vi "semLabV.vi"() -> ()   [LabVIEW 2021]
uses:
  <vilib>/userDefined/High Color/IMAQdx.ctl
  <vilib>/vision/driver/IMAQdx.llb/IMAQdx Camera Control Mode.ctl
  <vilib>/vision/driver/IMAQdx.llb/IMAQdx Acquisition Mode.ctl
  <vilib>/vision/driver/IMAQdx.llb/IMAQdx Buffer Number Mode.ctl
  <vilib>/myRIO/Instrument Drivers/Onboard IO/PWM/typedefs/PWM Reference.ctl
  <vilib>/myRIO/Common/Instrument Driver Framework/Utilities/typedefs/myRIO Generic Hardware Reference.ctl
  <vilib>/myRIO/Common/Instrument Driver Framework/Utilities/typedefs/Hardware Version Enum.ctl
  <vilib>/myRIO/Common/Instrument Driver Framework/Utilities/typedefs/myRIO v1.0 Reference.ctl
  <vilib>/myRIO/Common/Instrument Driver Framework/Utilities/typedefs/Generic FPGA Reference.ctl
  <vilib>/myRIO/Common/Instrument Driver Framework/myRIO v1.0/PWM/typedefs/PWM Channels Enum.ctl
  <vilib>/myRIO/Instrument Drivers/Onboard IO/PWM/typedefs/PWM Configuration.ctl
  <vilib>/userDefined/High Color/nirio_resource_hc.ctl
  <vilib>/myRIO/Common/Instrument Driver Framework/myRIO v1.0/PWM/vis/myRIO v1.1 Open PWM.vi
  <vilib>/myRIO/Common/Instrument Driver Framework/Utilities/vis/Validate Channels.vi
  <vilib>/myRIO/Common/Instrument Driver Framework/myRIO v1.0/PWM/vis/myRIO v1.0 Reserve PWM.vi
  <vilib>/myRIO/Instrument Drivers/Onboard IO/PWM/vis/Set Duty Cycle and Frequency.vi
  <vilib>/myRIO/Common/Instrument Driver Framework/myRIO v1.0/PWM/vis/myRIO v1.0 Close PWM.vi
  <vilib>/myRIO/Common/Instrument Driver Framework/myRIO v1.0/PWM/vis/myRIO v1.0 Build MUX Configuration PWM.vi
  <vilib>/myRIO/Common/Instrument Driver Framework/myRIO v1.0/Resource Manager/vis/myRIO v1.0 Reserve Channel List.vi
  <vilib>/myRIO/Common/Instrument Driver Framework/myRIO v1.0/PWM/vis/myRIO v1.0 Unreserve PWM.vi
  <vilib>/myRIO/Common/Instrument Driver Framework/myRIO v1.0/Resource Manager/vis/myRIO v1.0 Create Configuration List.vi
  <vilib>/myRIO/Common/Instrument Driver Framework/myRIO v1.0/Resource Manager/vis/myRIO v1.0 Reserve Channel.vi
  <vilib>/myRIO/Common/Instrument Driver Framework/myRIO v1.0/Resource Manager/vis/myRIO v1.0 Unreserve Channel.vi
  <vilib>/myRIO/Common/Instrument Driver Framework/myRIO v1.0/Resource Manager/vis/myRIO v1.0 Unreserve Channel List.vi
  <vilib>/myRIO/Common/Instrument Driver Framework/myRIO v1.0/Resource Manager/vis/myRIO v1.0 Build Mutex Name.vi
  <vilib>/Utility/VariantDataType/GetNumericInfo.vi
  <vilib>/Utility/error.llb/Error Cluster From Error Code.vi
  <vilib>/myRIO/Common/Instrument Driver Framework/myRIO v1.0/myRIO v1.1 Open.vi
  <vilib>/myRIO/Common/Instrument Driver Framework/Utilities/vis/IO Manager.vi
  <vilib>/myRIO/Common/Instrument Driver Framework/Utilities/vis/Configuration Manager.vi
  <vilib>/myRIO/Common/Instrument Driver Framework/myRIO v1.0/Resource Manager/vis/myRIO v1.0 Configure IO.vi
  <vilib>/myRIO/Common/Instrument Driver Framework/myRIO v1.0/myRIO v1.0 Close.vi
  <vilib>/myRIO/Common/Instrument Driver Framework/myRIO v1.0/PWM/vis/myRIO v1.0 Write PWM.vi
  <vilib>/myRIO/Common/Instrument Driver Framework/myRIO v1.0/PWM/vis/myRIO v1.0 Shutdown PWM.vi
  <vilib>/myRIO/Instrument Drivers/Onboard IO/PWM/vis/myRIO PWM Open.xnode
  <vilib>/vision/driver/NI_Vision_Acquisition_Software.lvlib
  <vilib>/vision/NI_Vision_Development_Module.lvlib
  <vilib>/myRIO/Instrument Drivers/Onboard IO/PWM/PWM.lvlib
panel:
  in  "Knob":dbl(knob) scale=0.0..180.0
  in  "error in 2":errorcluster
  out "Color Box":u32(colorbox)
  out "Colour Value":u32
  out "Circles Data":T1(array[cluster])
  in  "Min Radius":sgl=1.0 format="%.2f"
  in  "Max Radius":sgl=10.0 format="%.2f"
  in  "Settings":T2={"Objects"=0, "Threshold"=128, "Reject Border"=FALSE, "Fill Holes"=FALSE, "Min Object Size"=FALSE, "Min Size"=3, "Max Object Size"=FALSE, "Max Size"=100, "Show Search Area"=FALSE, "Show Center"=TRUE, "Show Bounding Box"=TRUE} {"Objects" items=["Bright Objects", "Dark Objects"]; "Threshold" min=1 max=999999999 step=1; "Max Size" min=1 max=999999999 step=1; "Min Size" min=1 max=999999999 step=1}
  out "circles":i32
  out "object":i32
  in  "error in (no error)":errorcluster
  in  "stop":bool
  out "Image":T3(plugin-control)
  in  "error in":errorcluster
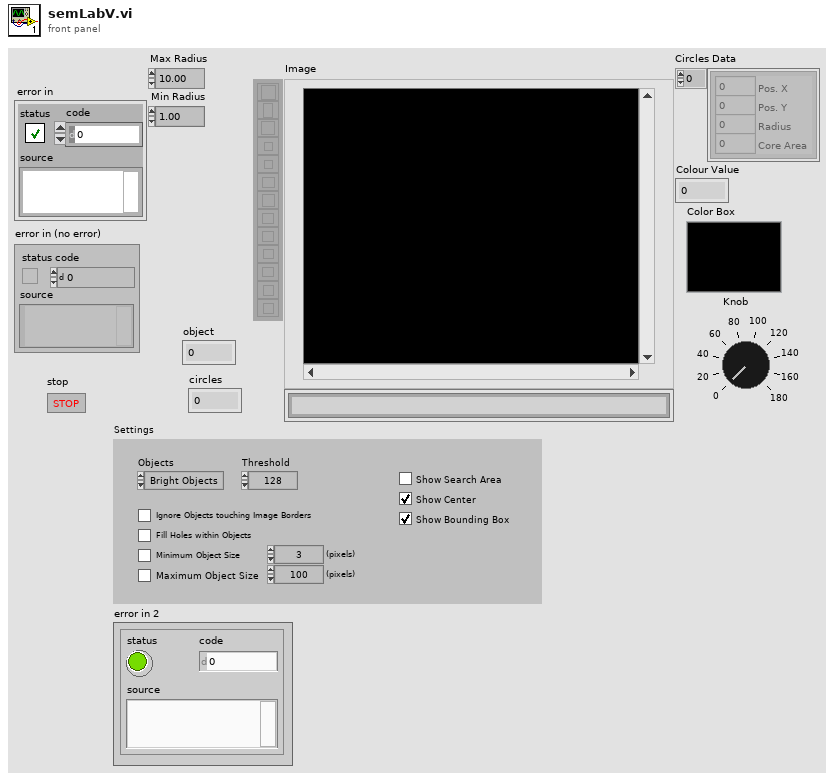
[diagram p1: front panel]
types:
  T1 = cluster{"Pos. X":i32, "Pos. Y":i32, "Radius":i32, "Core Area":i32}[]
  T2 = cluster{"Objects":u16, "Threshold":i32, "Reject Border":bool, "Fill Holes":bool, "Min Object Size":bool, "Min Size":i32, "Max Object Size":bool, "Max Size":i32, "Show Search Area":bool, "Show Center":bool, "Show Bounding Box":bool}
  T3 = typedef "IMAQ Image.ctl" = refnum<image>
  T4 = typedef "NI_Vision_Acquisition_Software.lvlib/IMAQdx Buffer Number Mode.ctl" = enum32{"Next", "Last", "Buffer Number", "Every", "Last New"}
  T5 = typedef "NI_Vision_Acquisition_Software.lvlib/IMAQdx Acquisition Mode.ctl" = enum32{"One Shot", "Continuous"}
  T6 = typedef "NI_Vision_Acquisition_Software.lvlib/IMAQdx Camera Control Mode.ctl" = enum32{"Controller", "Listener"}
  T7 = typedef "IMAQdx.ctl" = refnum<k21>
  T8 = typedef "PWM.lvlib/PWM Reference.ctl" = cluster{"myRIO Reference":T9, "PWM Channels Enum":T13, "PWM Configuration":T14}
  T9 = typedef "myRIO Generic Hardware Reference.ctl" = cluster{"myRIO Model":T10, "myRIO Hardware Reference":T11}
  T10 = typedef "Hardware Version Enum.ctl" = enum16{"Unknown", "myRIO-1900", "myRIO-1950", "roboRIO", "NI ELVIS RIO CM", "ELVIS III"}
  T11 = typedef "myRIO v1.0 Reference.ctl" = cluster{"Generic FPGA Reference":T12, "Allow multiple opens":bool}
  T12 = typedef "Generic FPGA Reference.ctl" = refnum<k20>
  T13 = typedef "PWM Channels Enum.ctl" = enum16{"Not Connected", "C/PWM0", "C/PWM1", "A/PWM0", "A/PWM1", "A/PWM2", "A/PWM3", "A/PWM4", "A/PWM5", "A/PWM6", "A/PWM7", "A/PWM8", "A/PWM9", "A/PWM10", "A/PWM11", "A/PWM12", "A/PWM13", "A/PWM14", "A/PWM15", "A/PWM16", "A/PWM17", "A/PWM18", "A/PWM19", "B/PWM0", "B/PWM1", "B/PWM2", "B/PWM3", "B/PWM4", "B/PWM5", "B/PWM6", "B/PWM7", "B/PWM8", "B/PWM9", "B/PWM10", "B/PWM11", "B/PWM12", "B/PWM13", "B/PWM14", "B/PWM15", "B/PWM16", "B/PWM17", "B/PWM18", "B/PWM19", "PWM/PWM0", "PWM/PWM1", "PWM/PWM2", "PWM/PWM3", "PWM/PWM4", "PWM/PWM5", "PWM/PWM6", "PWM/PWM7", "PWM/PWM8", "PWM/PWM9"}
  T14 = typedef "PWM.lvlib/PWM Configuration.ctl" = cluster{"Frequency":dbl, "Duty Cycle":dbl}
  T15 = typedef "Image Type" = u32
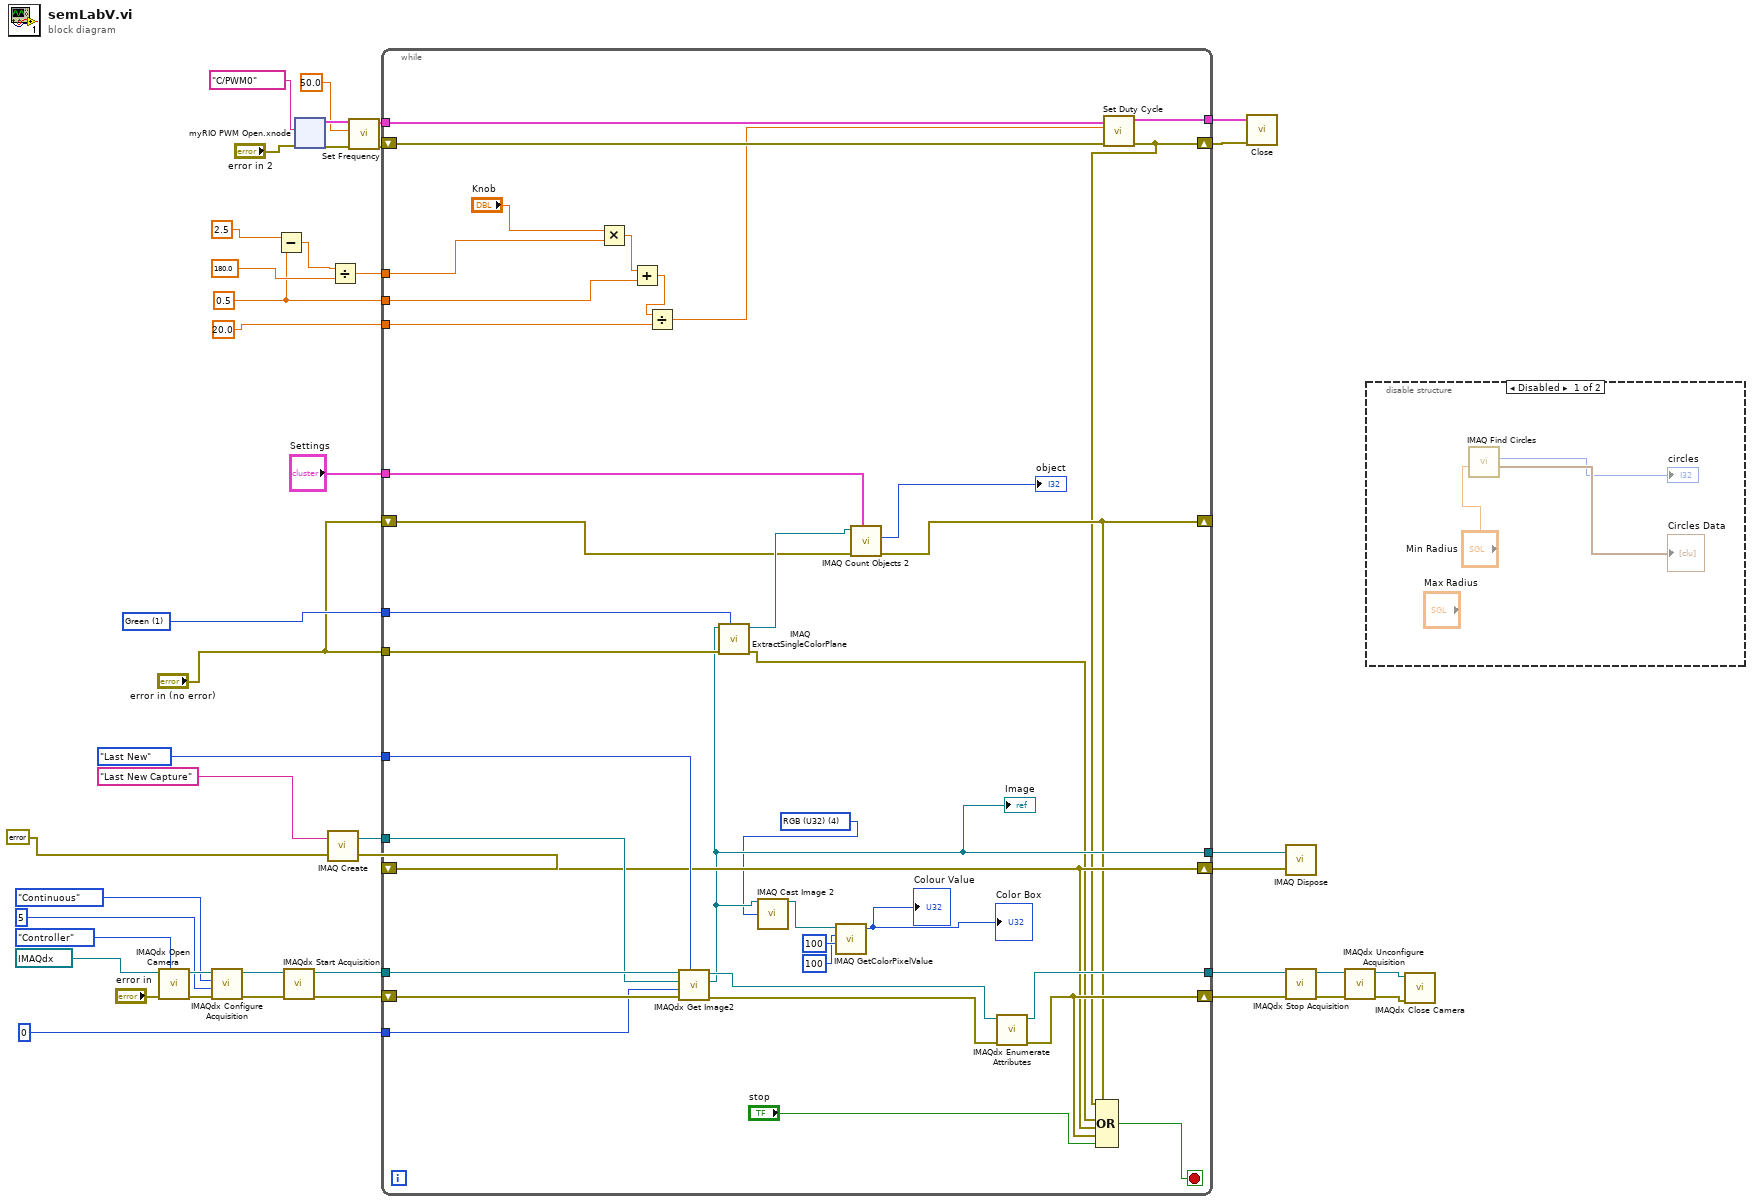
[diagram p0: block diagram]
diagram:
  w1 = 0.5
  w19 = 1 items=["Red", "Green", "Blue", "Hue", "Saturation", "Luminance", "Value", "Intensity"] ("Color Plane")
  n1 = call <vilib>:"IMAQdx Open Camera.vi"("Camera Control Mode"=IMAQdx_Camera_Control_Mode."Controller", "error in"="error in", "Session In"=T7 "cam0") -> ("error out"=w36:errorcluster, "Session Out"=w37:T7)  [unwired: 7 in]
  n2 = call <vilib>:"IMAQdx Configure Acquisition.vi"("error in"=w36, "Number of Buffers"=u32 5, "Continuous?"=IMAQdx_Acquisition_Mode."Continuous", "Session In"=w37) -> ("error out"=w43:errorcluster, "Session Out"=w42:T7)  [unwired: 6 in]
  n3 = Subtract(x=2.5, y=w1) -> (x-y=w6:dbl)
  n4 = call <vilib>:"IMAQdx Start Acquisition.vi"("error in"=w43, "Session In"=w42) -> ("error out"=w29:errorcluster, "Session Out"=w30:T7)  [unwired: 8 in]
  n5 = xnode "myRIO PWM Open.xnode"("error in (no error)"="error in 2", "Channel Name"=tag "C/PWM0") -> ("error out"=w14:errorcluster, "PWM Ref Out"=w13:T8)  [unwired: 1 in]
  n6 = call "IMAQ Create"("Image Name"="Last New Capture", "error in (no error)"=errorcluster {"status"=FALSE, "code"=0, "source"=""} ("error in")) -> ("New Image"=w26:T3, "error out"=w24:errorcluster)  [unwired: 3 in]
  n7 = Divide(x=w6, y=180.0) -> (x/y=w2:dbl)
  n8 = call <vilib>:"Set Frequency.vi"("error in (no error)"=w14, "Frequency [Hz]"=50.0, "PWM Ref In"=w13) -> ("error out"=w10:errorcluster, "PWM Ref Out"=w8:T8)  [unwired: 6 in]
  n9 = while {
    tunnel: w30 -> [w80]
    shift-right: [w65] -> w23
    shift-left: w29 -> [w79]
    tunnel: w26 -> [w78]
    shift-right: [w64] -> w25
    shift-left: w24 -> [w64]
    tunnel: [w59] -> w22
    tunnel: [w77] -> w21
    tunnel: u32 0 ("Buffer Number In") -> [w75]
    tunnel: "error in (no error)" -> [w74]
    tunnel: w19 -> [w73]
    shift-right: [w56] -> _
    shift-left: "error in (no error)" -> [w71]
    tunnel: IMAQdx_Buffer_Number_Mode."Last New" ("Buffer Number Mode (Next)") -> [w70]
    tunnel: "Settings" -> [w68]
    shift-right: [w51] -> w9
    shift-left: w10 -> [w54]
    tunnel: w8 -> [w53]
    tunnel: [w52] -> w7
    tunnel: w1 -> [w47]
    tunnel: 20.0 -> [w46]
    tunnel: w2 -> [w45]
    stop <- w67 stop-if-true
    w57 = T15 4 items=["Grayscale (U8)", "Grayscale (I16)", "Grayscale (SGL)", "Complex (CSG)", "RGB (U32)", "HSL (U32)", "RGB (U64)", "Grayscale (U16)"] ("Image Type")
    n10 = Multiply(x="Knob", y=w45) -> (x*y=w49:dbl)
    n11 = Add(x=w49, y=w47) -> (x+y=w48:dbl)
    n12 = Divide(x=w48, y=w46) -> (x/y=w44:dbl)
    n13 = call <vilib>:"IMAQdx Get Image2.vi"("Buffer Number Mode (Next)"=w70, "error in"=w79, "Buffer Number In"=w75, "Image In"=w78, "Session In"=w80) -> ("error out"=w76:errorcluster, "Image Out"=w59:T3, "Session Out"=w60:T7)  [unwired: 3 in, 1 out]
    "Image" <- w59
    n14 = call "IMAQ ExtractSingleColorPlane"("Color Plane"=w73, "error in (no error)"=w74, "Image Src"=w59) -> ("error out"=w55:errorcluster, "Image Dst Out"=w72:T3)  [unwired: 7 in]
    n15 = call "IMAQ Cast Image 2"("Image Src"=w59, "Image Type"=w57) -> ("Image Dst Out"=w58:T3)  [unwired: 12 in, 1 out]
    n16 = call "IMAQ GetColorPixelValue"("Y Coordinate"=100, "X Coordinate"=100, "Image"=w58) -> ("Pixel Value (U32)"=→"Colour Value" →"Color Box":u32)  [unwired: 1 in, 2 out]
    n17 = call "IMAQ Count Objects 2"("Settings"=w68, "error in (no error)"=w71, "Image"=w72) -> ("error out"=w56:errorcluster, "Number of Objects"=→"object":i32)  [unwired: 4 in, 3 out]
    n18 = call <vilib>:"IMAQdx Enumerate Attributes.vi"("error in"=w76, "Session In"=w60) -> ("error out"=w65:errorcluster, "Session Out"=w77:T7)  [unwired: 7 in, 1 out]
    n19 = call <vilib>:"Set Duty Cycle.vi"("error in (no error)"=w54, "Duty Cycle"=w44, "PWM Ref In"=w53) -> ("error out"=w51:errorcluster, "PWM Ref Out"=w52:T8)  [unwired: 6 in]
    n20 = Compound Arithmetic op=OR(w51, w56, w55, w64, w65, "stop") -> (w67:bool)
  }
  n21 = call <vilib>:"Close.vi"("error in (no error)"=w9, "PWM Ref In"=w7) -> ()  [unwired: 9 in, 1 out]
  n22 = call "IMAQ Dispose"("Image"=w22, "error in (no error)"=w25) -> ()  [unwired: 4 in, 1 out]
  n23 = call <vilib>:"IMAQdx Stop Acquisition.vi"("error in"=w23, "Session In"=w21) -> ("error out"=w39:errorcluster, "Session Out"=w40:T7)  [unwired: 8 in]
  n24 = call <vilib>:"IMAQdx Unconfigure Acquisition.vi"("error in"=w39, "Session In"=w40) -> ("error out"=w38:errorcluster, "Session Out"=w41:T7)  [unwired: 8 in]
  n25 = disable-structure shown="Disabled" {
    frame Disabled {
      n26 = call "IMAQ Find Circles"("Min Radius"="Min Radius") -> ("Circles Data"=→"Circles Data":T1, "Nb Circles"=→"circles":i32, "Max Radius"=w83:sgl)  [unwired: 6 in, 2 out]
    }
    frame Enabled {
    }
  }
  n27 = call <vilib>:"IMAQdx Close Camera.vi"("error in"=w38, "Session In"=w41) -> ()  [unwired: 9 in, 1 out]
